vi "DSA_Sync_Metrics.vi"() -> ()   [LabVIEW 2019]
uses:
  src/Instrument.DAQ/Typedefs/DAQ.Sampling.Sampling--Cluster.ctl
  src/Instrument.Lockin/Instrument.Lockin.lvclass
  src/Instrument.Lockin/Typedefs/Results Type--Enum.ctl
  src/Instrument.DAQ/Instrument.DAQ.lvclass
panel:
  out "Frequency (Hz)":dbl=13.0
  out "appended array":dbl[][](array[numeric])
  out "N":i32=97280
  out "XY Graph 3":cluster{dbl[], dbl[]}[](graph)
  in  "stop":bool
  out "Fs (Hz)":dbl=100.0
  out "XY Graph":cluster{i32[], dbl[]}[](graph)
  in  "f step":dbl=10000.0
  in  "f end":dbl=123456.0
  in  "f start":dbl=12345.0
  # "Sampling  frequency:"
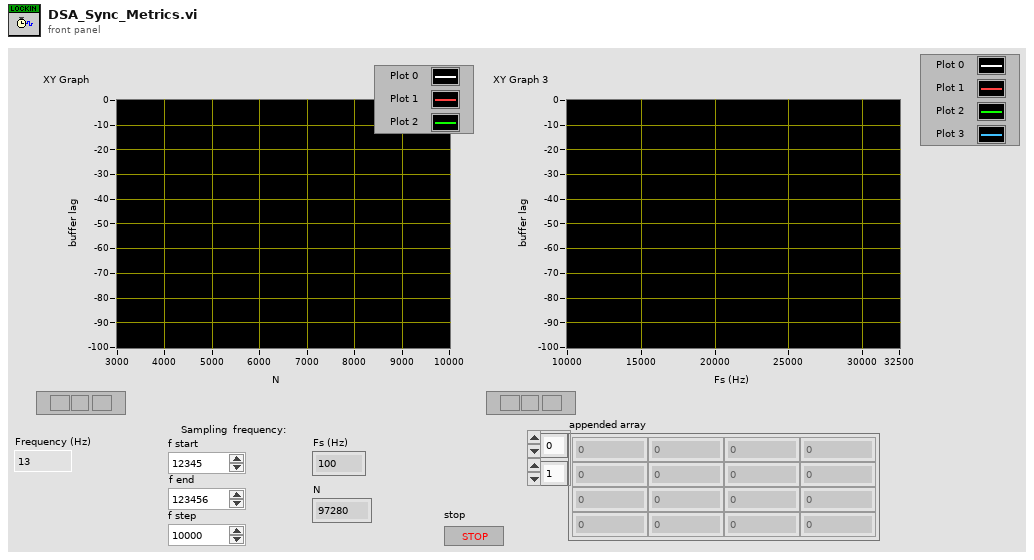
[diagram p1: front panel]
types:
  T1 = typedef "Instrument.Lockin.lvlib/Instrument.Lockin.lvclass/Results Type--Enum.ctl" = enum16{"X", "Y", "R", "Theta", "Mean"}
  T2 = typedef "Instrument.Lockin.lvlib/Instrument.DAQ.lvclass/DAQ.Sampling.Sampling--Cluster.ctl" = cluster{"Fs":dbl, "#s":i32}
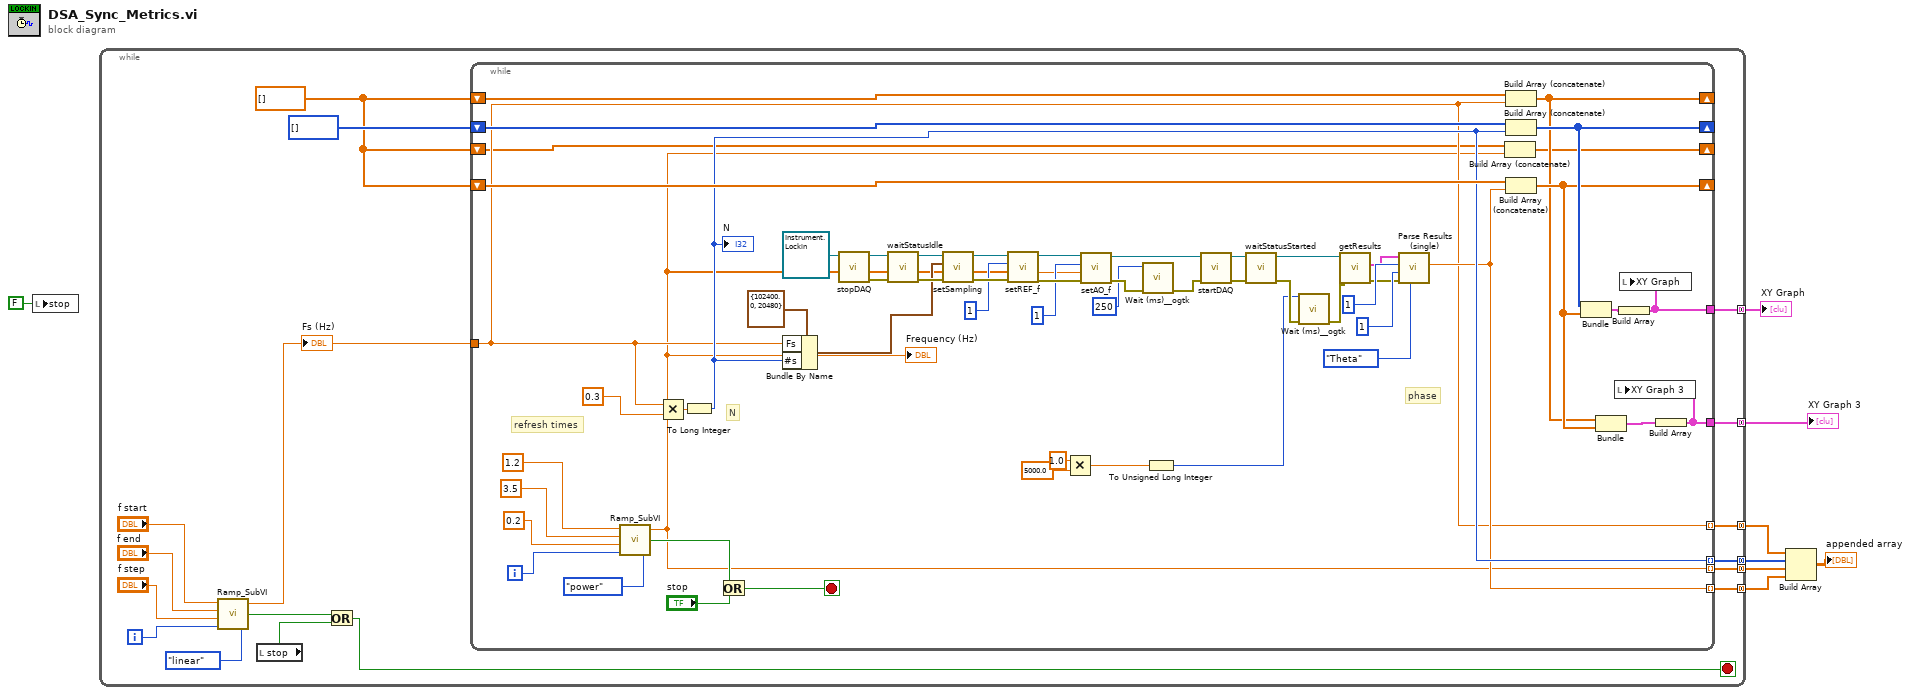
[diagram p0: block diagram]
diagram:
  n1 = local write "stop"(FALSE ("stop")) -> ()
  n2 = while {
    tunnel: [w21] -> w7 mode=concatenating
    tunnel: [w16] -> w6 mode=concatenating
    tunnel: [w14] -> w3 mode=concatenating
    tunnel: [w13] -> w4 mode=concatenating
    tunnel: [w12] -> w5 mode=concatenating
    tunnel: [w9] -> w1 mode=concatenating
    i -> [w24]
    stop <- w20 stop-if-true
    w10 = dbl[] []
    n3 = call <userlib>:"Ramp_SubVI.vi"("Enum"=enum16{"linear", "power"}."linear", "index"=w24, "step"="f step", "end"="f end", "start"="f start") -> ("Stop?"=w23:bool, "Numeric"=w11:dbl)
    "Fs (Hz)" <- w11
    n4 = local read "stop"() -> (w22:bool)
    n5 = Or(x=w23, y=w22) -> (x .or. y?=w20:bool)
    n6 = while {
      shift-right: [w71] -> _
      shift-left: w10 -> [w78]
      shift-right: [w68] -> _
      shift-left: w10 -> [w76]
      shift-right: [w72] -> _
      shift-left: i32[] [] -> [w77]
      tunnel: [w73] -> w21
      tunnel: w11 -> [w47]
      tunnel: [w69] -> w16
      tunnel: [w48] -> w14 mode=indexing
      tunnel: [w60] -> w13 mode=indexing
      tunnel: [w47] -> w12 mode=indexing
      shift-right: [w33] -> _
      shift-left: w10 -> [w32]
      tunnel: [w26] -> w9 mode=indexing
      i -> [w82]
      stop <- w75 stop-if-true
      # "N"
      # "phase"
      # "refresh times"
      n7 = call <userlib>:"Ramp_SubVI.vi"("Enum"=enum16{"linear", "power"}."power", "index"=w82, "step"=0.2 ("x"), "end"=3.5 ("x"), "start"=1.2 ("x")) -> ("Stop?"=w79:bool, "Numeric"=w26:dbl)
      "Frequency (Hz)" <- w26
      n8 = Multiply(x=w47, y=0.3 ("x")) -> (x*y=w57:dbl)
      n9 = To Long Integer(number=w57) -> (32bit integer=w60:i32)
      "N" <- w60
      n10 = Or(x=w79, y="stop") -> (x .or. y?=w75:bool)
      n11 = Bundle By Name(cluster=T2 {"Fs"=102400.0, "#s"=20480} ("Sampling"), "Fs"=w47, "#s"=w60) -> (w45:T2)
      n12 = call-dynamic "stopDAQ.vi"("Instrument.Lockin in"=refnum<class "Instrument.Lockin.lvclass"> refnum) -> ("error out"=w62:errorcluster, "Instrument.Lockin out"=w63:refnum<class "Instrument.Lockin.lvclass">)  [unwired: 9 in]
      n13 = call-dynamic "waitStatusIdle.vi"("error in (no error)"=w62, "Instrument.Lockin in"=w63) -> ("error out"=w59:errorcluster, "Instrument.Lockin out"=w58:refnum<class "Instrument.Lockin.lvclass">)  [unwired: 8 in]
      n14 = call-dynamic "setSampling.vi"("error in (no error)"=w59, "sampling"=w45, "Instrument.Lockin in"=w58) -> ("error out"=w38:errorcluster, "Instrument.Lockin out"=w37:refnum<class "Instrument.Lockin.lvclass">)  [unwired: 7 in]
      n15 = call-dynamic "setREF_f.vi"("error in (no error)"=w38, "Frequency (Hz)"=w26, "REF Channel"=1, "Instrument.Lockin in"=w37) -> ("error out"=w40:errorcluster, "Instrument.Lockin out"=w41:refnum<class "Instrument.Lockin.lvclass">)  [unwired: 6 in]
      n16 = Multiply(x=1.0, y=5000.0) -> (x*y=w56:dbl)
      n17 = call-dynamic "setAO_f.vi"("error in (no error)"=w40, "Frequency (Hz)"=w26, "AO Channel"=1, "Instrument.Lockin in"=w41) -> ("error out"=w31:errorcluster, "Instrument.Lockin out"=w43:refnum<class "Instrument.Lockin.lvclass">)  [unwired: 6 in]
      n18 = call <userlib>:"Wait (ms)__ogtk.vi"("error in (no error)"=w31, "milliseconds to wait"=u32 250) -> ("error out"=w29:errorcluster)  [unwired: 8 in, 1 out]
      n19 = To Unsigned Long Integer(number=w56) -> (unsigned 32bit integer=w28:u32)
      n20 = call-dynamic "startDAQ.vi"("error in (no error)"=w29, "Instrument.Lockin in"=w43) -> ("error out"=w35:errorcluster, "Instrument.Lockin out"=w44:refnum<class "Instrument.Lockin.lvclass">)  [unwired: 8 in]
      n21 = call-dynamic "waitStatusStarted.vi"("error in (no error)"=w35, "Instrument.Lockin in"=w44) -> ("error out"=w34:errorcluster, "Instrument.Lockin out"=w42:refnum<class "Instrument.Lockin.lvclass">)  [unwired: 8 in]
      n22 = call <userlib>:"Wait (ms)__ogtk.vi"("error in (no error)"=w34, "milliseconds to wait"=w28) -> ("error out"=w51:errorcluster)  [unwired: 8 in, 1 out]
      n23 = call-dynamic "getResults.vi"("error in (no error)"=w51, "Instrument.Lockin in"=w42) -> ("error out"=w50:errorcluster, "Results (Dictionary)"=w49:cluster{"key":string, "value":dbl}[])  [unwired: 6 in, 2 out]
      n24 = call "Parse Results (single).vi"("Type"=Results_Type--Enum."Theta", "error in (no error)"=w50, "Reference Channel"=1, "AI Channel"=1, "Results (Dictionary)"=w49) -> ("Data"=w48:dbl)  [unwired: 3 in, 3 out]
      n25 = Build Array (concatenate)(w32, w26) -> (w33:dbl[])
      n26 = Build Array (concatenate)(w76, w47) -> (w68:dbl[])
      n27 = Build Array (concatenate)(w77, w60) -> (w72:i32[])
      n28 = Build Array (concatenate)(w78, w48) -> (w71:dbl[])
      n29 = Bundle(w72, w71) -> (w74:cluster{i32[], dbl[]})  [unwired: 1 in]
      n30 = Bundle(w68, w71) -> (w70:cluster{dbl[], dbl[]})  [unwired: 1 in]
      n31 = Build Array(w74) -> (w73:cluster{i32[], dbl[]}[])
      n32 = local write "XY Graph"(w73) -> ()
      n33 = Build Array(w70) -> (w69:cluster{dbl[], dbl[]}[])
      n34 = local write "XY Graph 3"(w69) -> ()
    }
  }
  "XY Graph" <- w7
  "XY Graph 3" <- w6
  n35 = Build Array(w5, w4, w1, w3) -> (→"appended array":dbl[][])
